vi "DisabledSingle.vi"(8 "error in":errorcluster, 9 "Disabled":T1(ring), 10 "Control Label":string, 11 "UI Ref cluster in":T2) -> (0 "error out":errorcluster, 3 "UI Ref cluster out":T2)   [LabVIEW 2025, in "UI_Library.lvlib" / "UI_Library.lvclass"]
doc: "Enable\\Disable Control if found"
uses:
  UI_Library.lvclass
  Controls/UI_RefCluster.ctl
  <vilib>/Utility/Data Type/Type Definitions/Data Type.ctl
  UI_Library.lvlib
  <vilib>/Utility/Data Type/NI_Data Type.lvlib
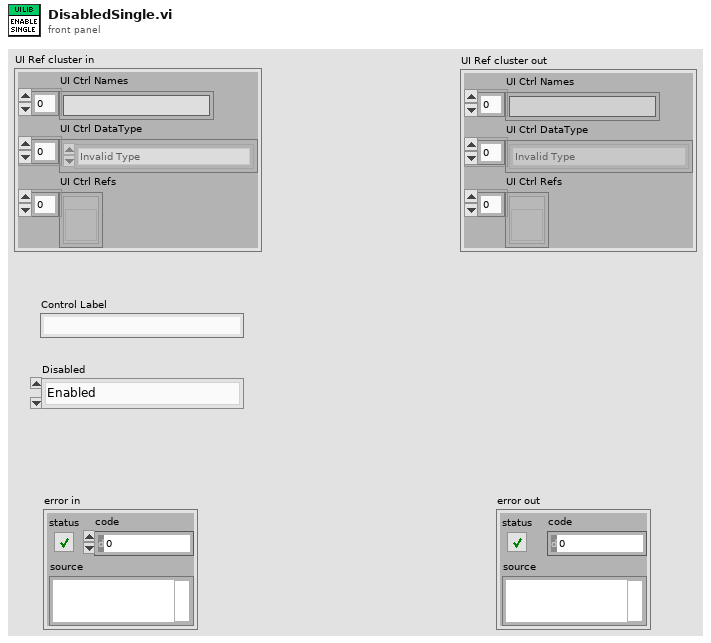
[diagram p1: front panel]
types:
  T1 = enum8{"Enabled", "Disabled", "Disabled and Grayed Out"}
  T2 = typedef "UI_Library.lvlib/UI_RefCluster.ctl" = cluster{"UI Ctrl Names":string[], "UI Ctrl DataType":T3[], "UI Ctrl Refs":refnum<vi>[]}
  T3 = typedef "NI_Data Type.lvlib/Data Type.ctl" = enum8{"Invalid Type", "Void", "I8", "I16", "I32", "I64", "U8", "U16", "U32", "U64", "Single Float", "Double Float", "Extended Float", "Single Complex", "Double Complex", "Extended Complex", "Enum U8", "Enum U16", "Enum U32", "Enum U64", "Single Float With Unit", "Double Float With Unit", "Extended Float With Unit", "Single Complex with Unit", "Double Complex with Unit", "Extended Complex with Unit", "Boolean", "String", "Path", "Picture", "Tag", "Array", "Cluster", "Variant", "LV Variant", "Waveform", "Timestamp", "Digital Waveform", "Digital Data", "ExpressData", "Refnum", "External Data", "VI", "Poly VI", "LabVIEW Class Instance", "Fixed Point", "Set Collection", "Map Collection"}
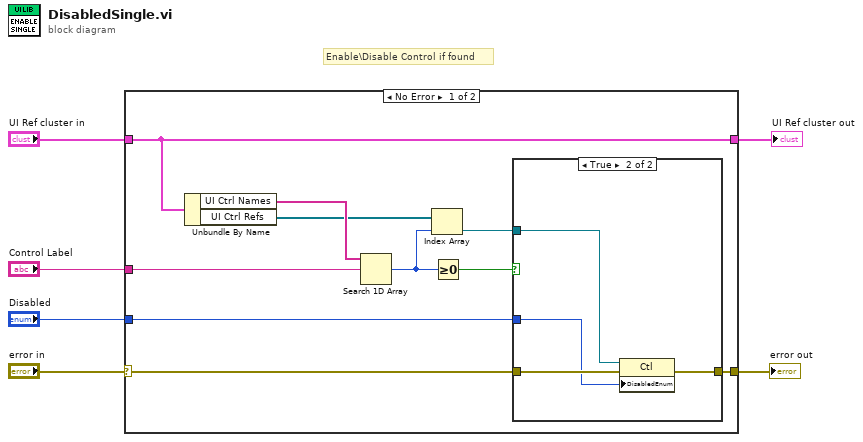
[diagram p0: block diagram]
diagram:
  # "Enable\\Disable Control if found"
  n1 = case shown="No Error" "error in" {
    selector: "error in" -> [w10 w23]
    tunnel: [w9 w23] -> w6
    tunnel: "Control Label" -> [w15 _]
    tunnel: [w8 w22] -> w3
    tunnel: "UI Ref cluster in" -> [w8 w22]
    tunnel: "Disabled" -> [w7 _]
    frame No Error {
      n2 = Unbundle By Name(w8) -> ("UI Ctrl Names"=w16:string[], "UI Ctrl Refs"=w13:refnum<vi>[])
      n3 = Search 1D Array(1D array=w16, element=w15) -> (index of element=w12:i32)  [unwired: 1 in]
      n4 = Index Array(array=w13, index=w12) -> (element=w11:refnum<vi>)
      n5 = Greater Or Equal To 0?(x=w12) -> (x >= 0?=w14:bool)
      n6 = case shown="True" w14 {
        tunnel: w11 -> [_ w21]
        tunnel: w10 -> [w17 w19]
        tunnel: [w17 w20] -> w9
        tunnel: w7 -> [_ w18]
        frame False {
        }
        frame True {
          n7 = property class="Ctl"(reference=w21, error in=w19, "DisabledEnum"=w18) -> (error out=w20:errorcluster)  [unwired: 1 out]
        }
      }
    }
    frame Error {
    }
  }
  "error out" <- w6
  "UI Ref cluster out" <- w3
